vi "Exercise 5.1 - Shared Variable.vi"() -> ()   [LabVIEW 2024]
panel:
  in  "Led Switch for 2nd loop":bool
  in  "Led Switch":bool
  in  "stop":bool
  out "Boolean 2":bool
  out "Boolean":bool
  # "LED values and stop two loops \nwith one control"
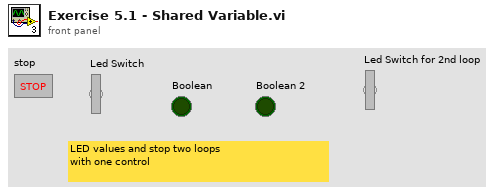
[diagram p1: front panel]
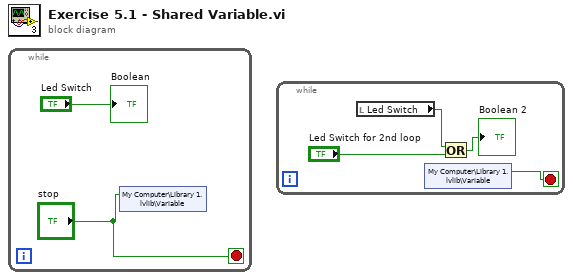
[diagram p0: block diagram]
diagram:
  n1 = while {
    stop <- "stop" stop-if-true
    n2 = shared-variable "My Computer\\Library 1.lvlib\\Variable"("stop") -> ()  [unwired: 1 in, 1 out]
    "Boolean" <- "Led Switch"
  }
  n3 = while {
    stop <- w3 stop-if-true
    n4 = local read "Led Switch"() -> (w6:bool)
    n5 = shared-variable "My Computer\\Library 1.lvlib\\Variable"() -> (w3:bool)  [unwired: 1 in, 1 out]
    n6 = Or(x=w6, y="Led Switch for 2nd loop") -> (x .or. y?=→"Boolean 2":bool)
  }
